vi "initialize timing source.vi"(8 "error in":errorcluster, 11 "timing source in":refnum<class "ms timing source.lvclass">) -> (0 "error out":errorcluster, 3 "timing source out":refnum<class "ms timing source.lvclass">)   [LabVIEW 2013, in "ms timing source.lvclass"]
doc: "An interface for initializing a timing source. In many cases this may be a no-op. There is no expectation about when this function should be called, but it must be called before entering the loop to be timed."
uses:
  ms timing source.lvclass
  ms timing source.lvclass/ms timing source.ctl
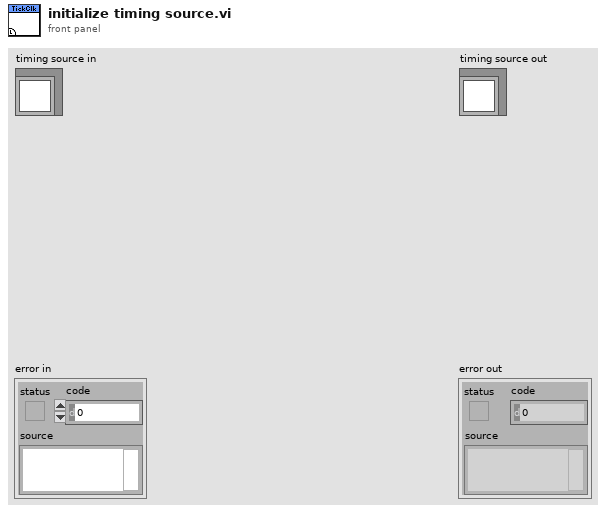
[diagram p1: front panel]
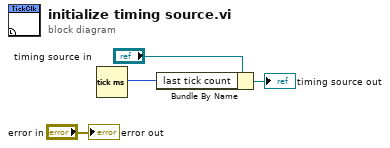
[diagram p0: block diagram]
diagram:
  n1 = Tick Count (ms)() -> (millisecond timer value=w1:u32)
  n2 = Bundle By Name(cluster="timing source in", "last tick count"=w1) -> (→"timing source out":refnum<class "ms timing source.lvclass">)
  "error out" <- "error in"
